vi "Set Contact Template Variables.vi"(8 "error in (no error)":errorcluster, 9 "Index (none)":i32=-1, 10 "Cluster":T1, 11 "LabVIEW Web Service Request":refnum<class "Web Request.lvclass">) -> (0 "error out":errorcluster, 3 "LabVIEW Web Service Request out":refnum<class "Web Request.lvclass">)   [LabVIEW 2014]
doc: "This VI sets all of the ESP variables for a single contact so it can be output from an ESP script."
uses:
  <vilib>/wsapi/Web Request.lvclass
  <vilib>/wsapi/class/subVIs/Set Many String ESP Variables.vi
  <vilib>/wsapi/class/subVIs/Set Integer ESP Variable.vi
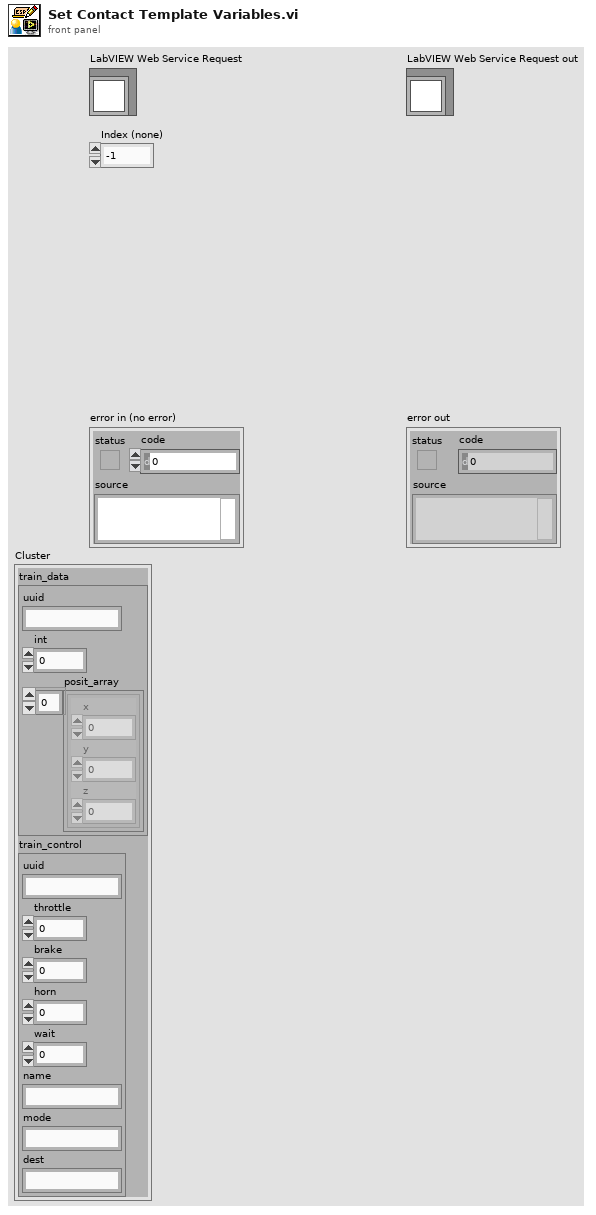
[diagram p1: front panel]
types:
  T1 = cluster{"train_data":cluster{"uuid":string, "int":i32, "posit_array":cluster{"x":dbl, "y":dbl, "z":dbl}[]}, "train_control":cluster{"uuid":string, "throttle":dbl, "brake":dbl, "horn":dbl, "wait":dbl, "name":string, "mode":string, "dest":string}}
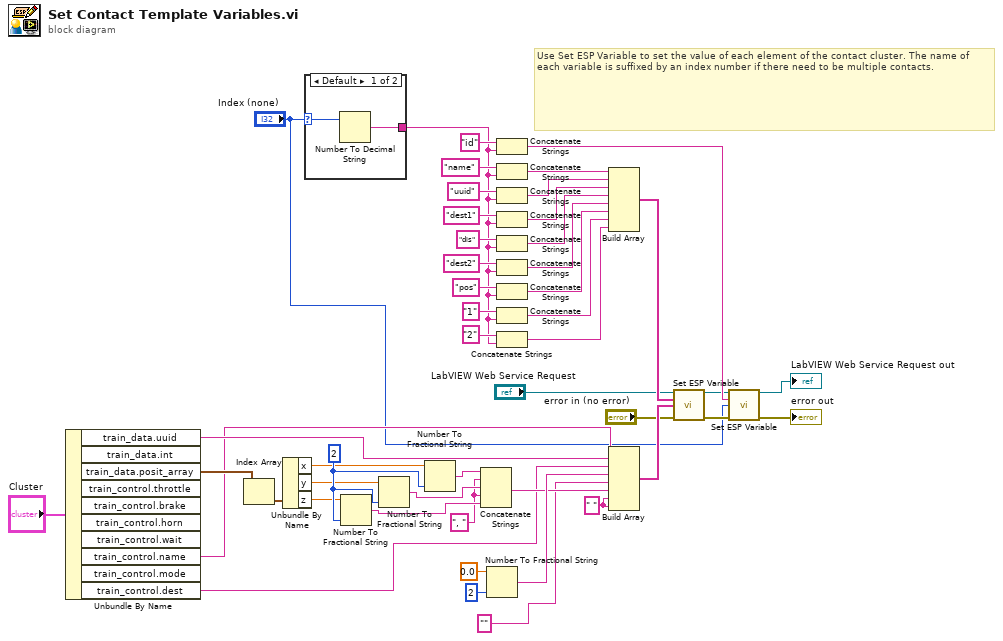
[diagram p0: block diagram]
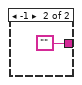
[diagram p2: hidden frame]
diagram:
  w13 = ", " ("string")
  w20 = i16 2 ("precision (6)")
  w19 = " " ("element")
  # "Use Set ESP Variable to set the value of each element of the contact cluster. The name of each variable is suffixed by an index number if there need to be multiple contacts."
  n1 = Unbundle By Name("Cluster") -> ("train_data.uuid"=w4:string, "train_data.posit_array"=w7:cluster{"x":dbl, "y":dbl, "z":dbl}[], "train_control.name"=w3:string, "train_control.dest"=w2:string)  [unwired: 6 out]
  n2 = Index Array(array=w7) -> (element=w12:cluster{"x":dbl, "y":dbl, "z":dbl})  [unwired: 1 in]
  n3 = Unbundle By Name(w12) -> ("x"=w11:dbl, "y"=w10:dbl, "z"=w9:dbl)
  n4 = case shown="Default" "Index (none)" {
    selector: "Index (none)" -> [w49 _]
    tunnel: [w50 ""] -> w37
    frame Default {
      n5 = Number To Decimal String(number=w49) -> (decimal integer string=w50:string)  [unwired: 1 in]
    }
    frame -1 {
    }
  }
  n6 = Number To Fractional String(number=w9, precision (6)=w20) -> (F-format string=w14:string)  [unwired: 2 in]
  n7 = Number To Fractional String(number=w10, precision (6)=w20) -> (F-format string=w15:string)  [unwired: 2 in]
  n8 = Number To Fractional String(number=w11, precision (6)=w20) -> (F-format string=w21:string)  [unwired: 2 in]
  n9 = Concatenate Strings(w21, w13, w15, w13, w14) -> (w16:string)
  n10 = Number To Fractional String(number=0.0, precision (6)=i16 2) -> (F-format string=w17:string)  [unwired: 2 in]
  n11 = Concatenate Strings("id" ("string"), w37) -> (w36:string)
  n12 = Concatenate Strings("name" ("string"), w37) -> (w35:string)
  n13 = Concatenate Strings("uuid" ("string"), w37) -> (w34:string)
  n14 = Concatenate Strings("dest1" ("string"), w37) -> (w33:string)
  n15 = Concatenate Strings("dis" ("string"), w37) -> (w32:string)
  n16 = Concatenate Strings("dest2" ("string"), w37) -> (w31:string)
  n17 = Concatenate Strings("pos" ("string"), w37) -> (w30:string)
  n18 = Concatenate Strings("1" ("string"), w37) -> (w29:string)
  n19 = Concatenate Strings("2" ("string"), w37) -> (w28:string)
  n20 = Build Array(w35, w34, w33, w32, w31, w30, w29, w28) -> (w27:string[])
  n21 = Build Array(w3, w4, w2, w17, "" ("Desination"), w16, w19, w19) -> (w26:string[])
  n22 = call-poly <vilib>:"Set ESP Variable.vi"("LabVIEW Web Service Request"="LabVIEW Web Service Request", "keys"=w27, "values"=w26, "error in (no error)"="error in (no error)") -> ("LabVIEW Web Service Request out"=w24:refnum<class "Web Request.lvclass">, "error out"=w25:errorcluster)  [unwired: 10 in]
  n23 = call-poly <vilib>:"Set ESP Variable.vi"("LabVIEW Web Service Request"=w24, "key"=w36, "value"="Index (none)", "error in (no error)"=w25) -> ("LabVIEW Web Service Request out"=→"LabVIEW Web Service Request out":refnum<class "Web Request.lvclass">, "error out"=→"error out":errorcluster)  [unwired: 10 in]
